vi "WaveformDAQ_tb3.vi"() -> ()   [LabVIEW 2018]
uses:
  <instrlib>/Agilent 33XXX Series/Agilent 33XXX Series.lvlib
panel:
  out "N Samples":dbl
  in  "Time":dbl
  in  "Sample rate":enum16{"1KHz", "10KHz", "100KHz", "1MHz"}(ring)
  out "Waveform Graph":dynamicdata(graph)
  in  "stop":bool
  in  "Frequency (1000 Hz)":dbl=1000.0
  in  "Waveform Function (1: Sine)":u16(ring)=1 items=["DC", "Sine", "Square", "Triangle", "Ramp", "Pulse", "Noise", "Sinc", "Negative Ramp", "Exponential Rise", "Exponential Fall", "Cardiac"]
  in  "Serial Configuration":T1={"Baud Rate"=9600, "Parity"=0, "Data Bits"=8, "Flow Control"=4} {"Flow Control" items=["None", "XON/XOFF", "RTS/CTS", "XON/XOFF & RTS/CTS", "DTR/DSR", "XON/XOFF & DTR/DSR"]; "Data Bits" items=["7"=7, "8"=8]; "Parity" items=["None", "Odd", "Even", "Mark", "Space"]; "Baud Rate" items=["300"=300, "600"=600, "1200"=1200, "2400"=2400, "4800"=4800, "9600"=9600, "19200"=19200]}
  in  "DC Offset (0.00 V)":dbl
  in  "Amplitude (1 Vpp)":dbl=1.0
  in  "VISA resource name":refnum<visa-resource-name>
  # "This VI is a stand-along DAQ testbench.  \nThis program \n1. set the Agilent to produce the required waveform,\n2. use the DAQ device to acquire the output form the sync port. \n3. Output the signal to the front panel."
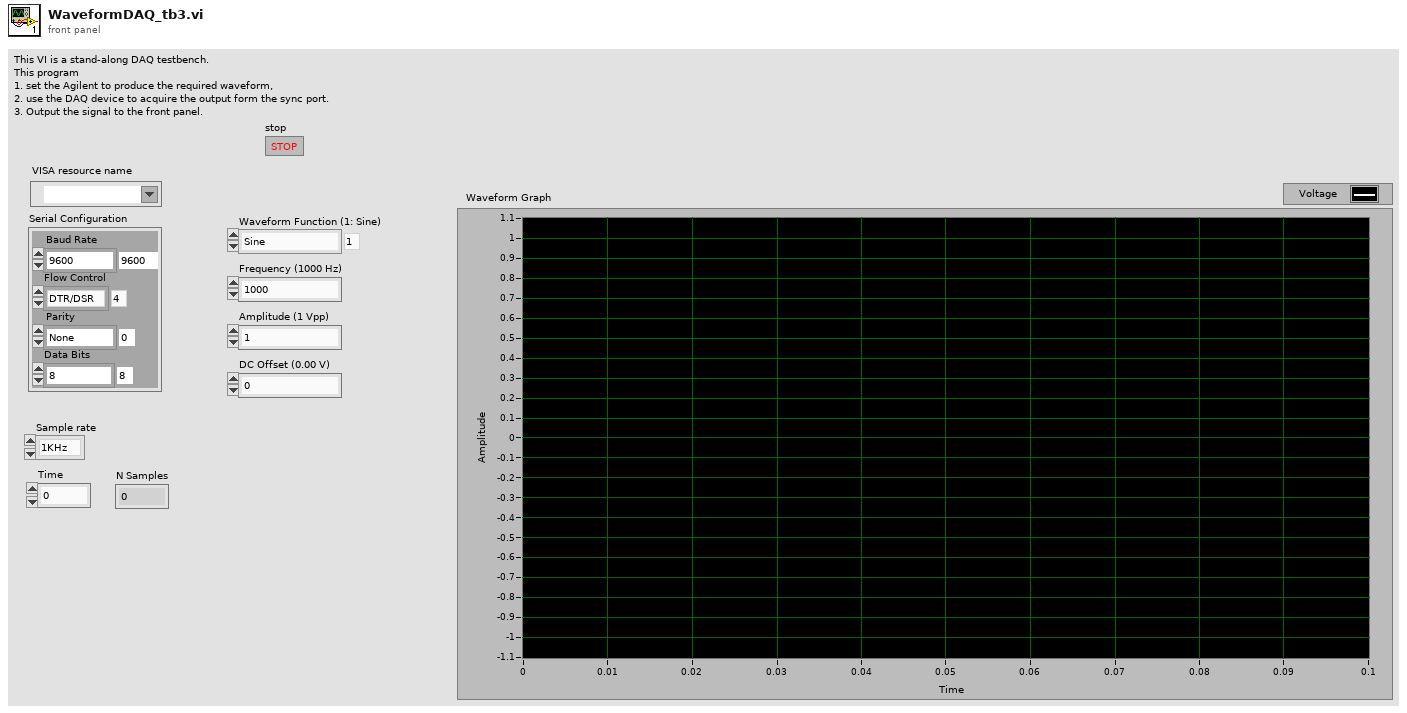
[diagram p1: front panel]
types:
  T1 = cluster{"Baud Rate":u32, "Parity":u16, "Data Bits":u16, "Flow Control":u16}
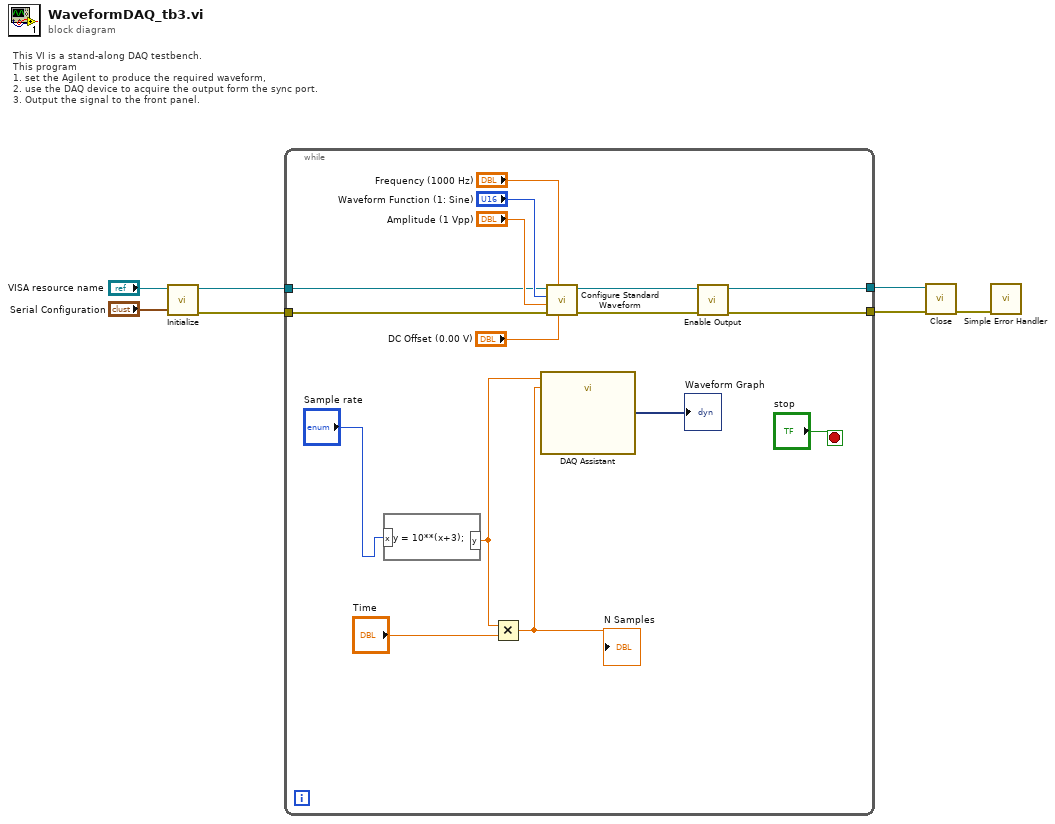
[diagram p0: block diagram]
diagram:
  # "This VI is a stand-along DAQ testbench.  \nThis program \n1. set the Agilent to produce the required waveform,\n2. use the DAQ device to acquire the output form the sync port. \n3. Output the signal to the front panel."
  n1 = call <instrlib>:"Initialize.vi"("Serial Configuration"="Serial Configuration", "VISA resource name"="VISA resource name") -> ("error out"=w2:errorcluster, "VISA resource name out"=w1:refnum<visa-resource-name>)  [unwired: 8 in]
  n2 = while {
    tunnel: [w13] -> w4
    tunnel: [w14] -> w3
    tunnel: w2 -> [w16]
    tunnel: w1 -> [w15]
    stop <- "stop" stop-if-true
    n3 = formula code="y = 10**(x+3);"("x"="Sample rate") -> ("y"=w10:dbl)
    n4 = Multiply(x=w10, y="Time") -> (x*y=w8:dbl)
    "N Samples" <- w8
    n5 = call "DAQ Assistant"("rate"=w10, "number of samples"=w8) -> ("data"=→"Waveform Graph":dynamicdata)  [unwired: 15 in, 2 out]
    n6 = call <instrlib>:"Configure Standard Waveform.vi"("DC Offset (0.00 V)"="DC Offset (0.00 V)", "Frequency (1000 Hz)"="Frequency (1000 Hz)", "error in (no error)"=w16, "Amplitude (1)"="Amplitude (1 Vpp)", "Waveform Function (1: Sine)"="Waveform Function (1: Sine)", "VISA resource name"=w15) -> ("error out"=w21:errorcluster, "VISA resource name out"=w20:refnum<visa-resource-name>)  [unwired: 4 in]
    n7 = call <instrlib>:"Enable Output.vi"("error in (no error)"=w21, "VISA resource name"=w20) -> ("error out"=w14:errorcluster, "VISA resource name out"=w13:refnum<visa-resource-name>)  [unwired: 8 in]
  }
  n8 = call <instrlib>:"Close.vi"("error in (no error)"=w3, "VISA resource name"=w4) -> ("error out"=w6:errorcluster)  [unwired: 9 in]
  n9 = call <vilib>:"Simple Error Handler.vi"("error in (no error)"=w6) -> ()  [unwired: 4 in, 5 out]
